vi "NavigationOffensive.vi"(8 "error in (no error)":errorcluster, 11 "Game in":refnum<class "Game.lvclass">) -> (0 "error out":errorcluster, 2 "NaN?":bool, 3 "Game out":refnum<class "Game.lvclass">)   [LabVIEW 2020, in "Game.lvclass"]
uses:
  Game.lvclass
  Ally_class/Ally.lvclass
  Parameters_class/Parameters.lvclass
panel:
  in  "GoTo Navigation":bool
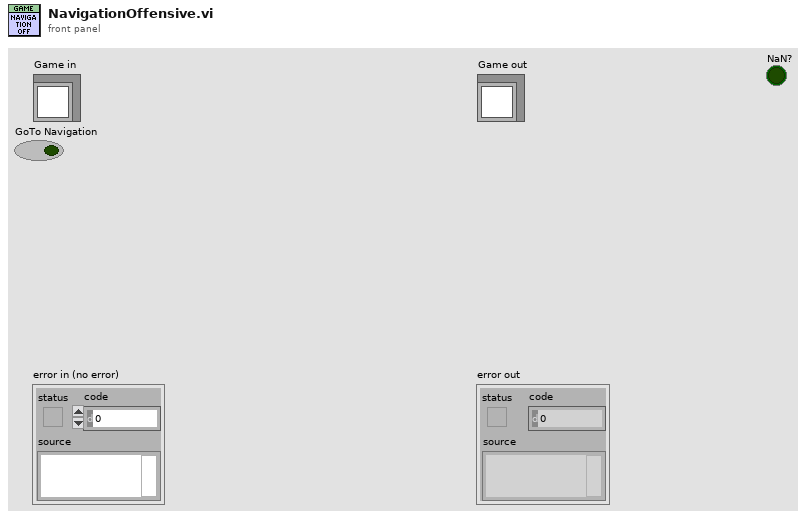
[diagram p1: front panel]
types:
  T1 = cluster{"(Kc)":dbl, "(Ti, min)":dbl, "(Td, min)":dbl}
  T2 = typedef "AI Input.ctl" = cluster{"our_robots":T3[], "enemy_robots":T3[], "balls":T10[], "geometry":T11, "IA Judge":T12, "Received Timestamp":timestamp, "Events":T14}
  T3 = typedef "AI Robot.ctl" = cluster{"id":u32, "function":T4, "x":dbl, "y":dbl, "orientation":dbl, "v_tangent":dbl, "v_normal":dbl, "v_ang":dbl, "kick_x":dbl, "kick_z":dbl, "dribble":bool, "Timestamp":timestamp, "estimatives":T5, "dest_x_kick":dbl, "dest_y_kick":dbl, "Gap Coord":dbl[], "States":T6, "Path ":dbl[][], "Path  Smooth":dbl[][], "Dest":T7, "vx_desired":dbl, "vy_desired":dbl, "slowBehavior":bool, "VSSStates":T9}
  T4 = typedef "Functions Enum.ctl" = enum16{"2nd Striker", "Attacker", "Goalie", "Defender", "Striker", "Goto 0", "Dummy", "Kicker", "ZigZag 0", "ZigZag 1", "ZigZag 2", "ZigZag 3", "ZigZag 4", "ZigZag 5", "ZigZag 6", "ZigZag 7", "ZigZag 8", ""}
  T5 = typedef "estimatives.ctl" = cluster{"est_v_tangent":dbl, "est_v_normal":dbl, "est_vx":dbl, "est_vy":dbl, "Pos Robot Est":dbl[], "est_v_ang":dbl}
  T6 = typedef "AttackerStates.ctl" = enum16{"Pass", "GoToTangent", "BallGetting", "GoToKick", ""}
  T7 = typedef "PathDests.ctl" = T8[]
  T8 = typedef "PathDest.ctl" = cluster{"dest_x":dbl, "dest_y":dbl, "dest_orientation":dbl, "dest_vel":dbl}
  T9 = typedef "VSSAttackerStates.ctl" = enum16{"Pass", "GoToTangent", "BallGetting", "GoToKick", "Rotate anti-clockwise", "Rotate Clockwise", ""}
  T10 = typedef "AI Ball.ctl" = cluster{"x":dbl, "y":dbl, "timestamp":timestamp, "Vel_x":dbl, "Vel_y":dbl, "Pos Bola Est":dbl[], "Valid":bool, "z":dbl, "Vel_z":dbl}
  T11 = typedef "Field Size.ctl" = cluster{"line_width":u32, "field_length":u32, "field_width":u32, "boundary_width":u32, "referee_width":u32, "goal_width":u32, "goal_depth":u32, "goal_wall_width":u32, "center_circle_radius":u32, "defense_radius":u32, "defense_stretch":u32, "free_kick_from_defense_dist":u32, "penalty_spot_from_field_line_dist":u32, "penalty_line_from_spot_dist":u32}
  T12 = typedef "AI Judge.ctl" = cluster{"stage":string, "command":string, "our_goalie_id":dbl, "enemy_goalie_id":dbl, "command enum":T13, "Time":enum16{"Azul", "Amarelo"}}
  T13 = typedef "Command Enum.ctl" = enum16{"Halt", "Stop", "Force Start", "PKA Normal Start", "Prepare Kickoff Ally", "PKE Normal Start", "Prepare Kickoff Enemy", "Prepare Penalty Ally", "PPA Normal Start", "Prepare Penalty Enemy", "PPE Normal Start", "Direct Free Enemy", "Direct Free Ally", "Indirect Free Enemy", "Indirect Free Ally", "Timeout Enemy", "Timeout Ally", "Goal Enemy", "Goal Ally", "Ball Placement Enemy", "Ball Placement Ally", "Normal Half Time", "Extra Time Break", "Extra Half Time", "None", "Post Game"}
  T14 = typedef "Events.ctl" = cluster{"Touch":bool, "Ball out":bool, "id touch":dbl, "Ball out of \nVision":bool, "Ball inside \nGoalie area":bool, "Robot not responding":bool, "Robots responding status":dbl[], "Enemy Ball \nPossession":bool, "Pass State":bool, "id end of pass":dbl, "Kick":bool, "Id ini Possession":dbl, "Ball Possesion":bool, "Id Possesion":dbl, "Direct Kick":bool, "2nd Strk Ativo":bool}
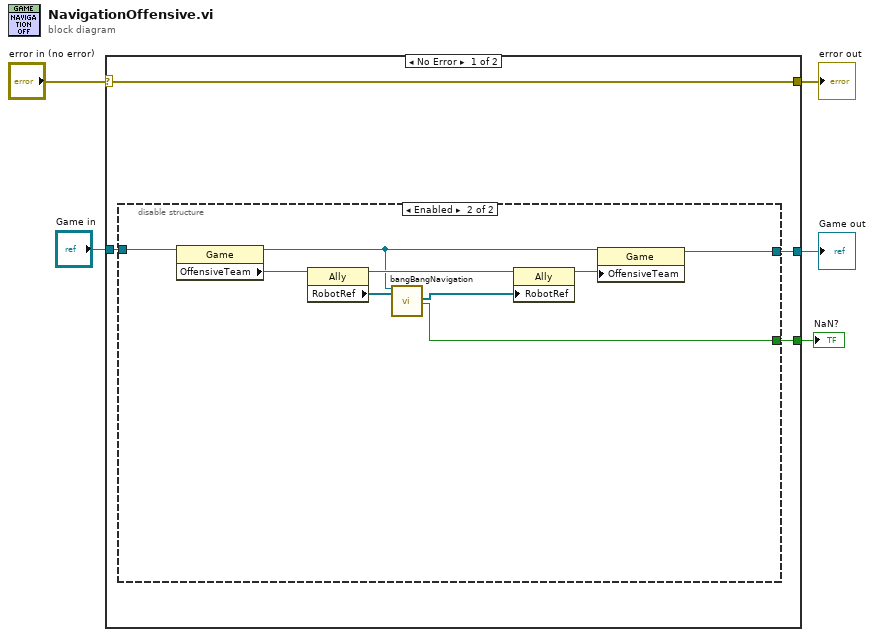
[diagram p0: block diagram]
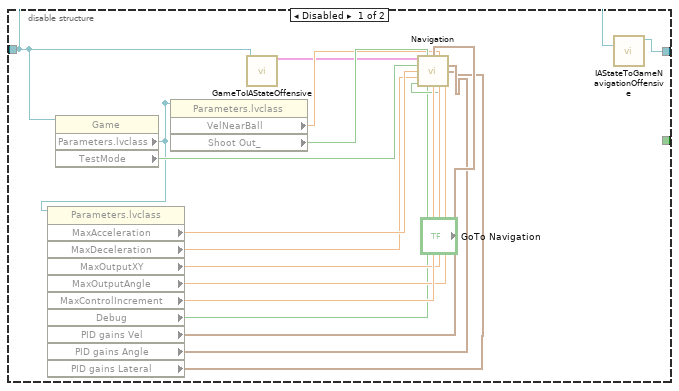
[diagram p2: hidden frame]
diagram:
  n1 = case shown="No Error" "error in (no error)" {
    selector: "error in (no error)" -> [w8 w37]
    tunnel: [w8 w37] -> w4
    tunnel: [w9 w36] -> w2
    tunnel: "Game in" -> [w7 w36]
    tunnel: [w6 _] -> w1
    frame No Error {
      n2 = disable-structure shown="Enabled" {
        disable-tunnel: [w26 w29] -> w9
        disable-tunnel: w7 -> [w11 w28]
        disable-tunnel: [_ w30] -> w6
        frame Disabled {
          n3 = property class="Game"(reference=w11) -> ("Parameters.lvclass"=w10:refnum<class "Parameters.lvclass">, "TestMode"=w17:bool)  [unwired: 1 in, 2 out]
          n4 = property class="Parameters.lvclass"(reference=w10) -> ("MaxAcceleration"=w25:dbl, "MaxDeceleration"=w24:dbl, "MaxOutputXY"=w22:dbl, "MaxOutputAngle"=w21:dbl, "MaxControlIncrement"=w23:dbl, "Debug"=w19:bool, "PID gains Vel"=w18:T1, "PID gains Angle"=w14:cluster{"(Kc)":dbl, "(Ki)":dbl, "(Kd)":dbl}, "PID gains Lateral"=w13:cluster{"(Kc)":dbl, "(Ki)":dbl, "(Kd)":dbl})  [unwired: 1 in, 2 out]
          n5 = property class="Parameters.lvclass"(reference=w10) -> ("VelNearBall"=w15:dbl, "Shoot Out_"=w16:bool)  [unwired: 1 in, 2 out]
          n6 = call-dynamic "GameToIAStateOffensive.vi"("Game in"=w11) -> ("IA State out"=w12:T2)  [unwired: 6 in, 4 out]
          n7 = call "Navigation.vi"("IA State Output in"=w12, "Penalty Shoot Out?"=w16, "PID gains Vel"=w18, "VelNearBall"=w15, "Test Mode"=w17, "PID gains Angle"=w14, "a1"=w25, "PID gains Lateral"=w13, "a3"=w24, "GoTo Navigation"="GoTo Navigation", "Debug"=w19, "output inc"=w23, "output xy"=w22, "output angle"=w21) -> ()  [unwired: 1 in, 1 out]
          n8 = call "IAStateToGameNavigationOffensive.vi"("Game in"=w11) -> ("Game out"=w26:refnum<class "Game.lvclass">)  [unwired: 9 in, 1 out]
        }
        frame Enabled {
          n9 = property class="Game"(reference=w28) -> (reference out=w27:refnum<class "Game.lvclass">, "OffensiveTeam"=w35:refnum<class "Ally.lvclass">)  [unwired: 1 in, 1 out]
          n10 = property class="Ally"(reference=w35) -> (reference out=w33:refnum<class "Ally.lvclass">, "RobotRef"=w34:refnum<class "Robot.lvclass">[])  [unwired: 1 in, 1 out]
          n11 = call "bangBangNavigation.vi"("Game"=w27, "RobotRef"=w34) -> ("RoboRef"=w32:refnum<class "Robot.lvclass">[], "NaN?"=w30:bool)  [unwired: 15 in, 1 out]
          n12 = property class="Ally"(reference=w33, "RobotRef"=w32) -> (reference out=w31:refnum<class "Ally.lvclass">)  [unwired: 1 in, 1 out]
          n13 = property class="Game"(reference=w27, "OffensiveTeam"=w31) -> (reference out=w29:refnum<class "Game.lvclass">)  [unwired: 1 in, 1 out]
        }
      }
    }
    frame Error {
    }
  }
  "error out" <- w4
  "Game out" <- w2
  "NaN?" <- w1
